vi "Error Converter (ErrCode or Status).vi"(8 "error in (no error)":errorcluster, 11 "error code":i32) -> (0 "error out":errorcluster)   [LabVIEW 2012, in "clearvolume.lvlib"]
uses:
  clearvolume.lvlib
panel:
  in  "string":string="This error is returned by the shared library function."
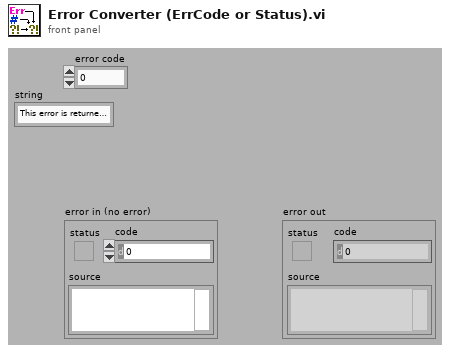
[diagram p1: front panel]
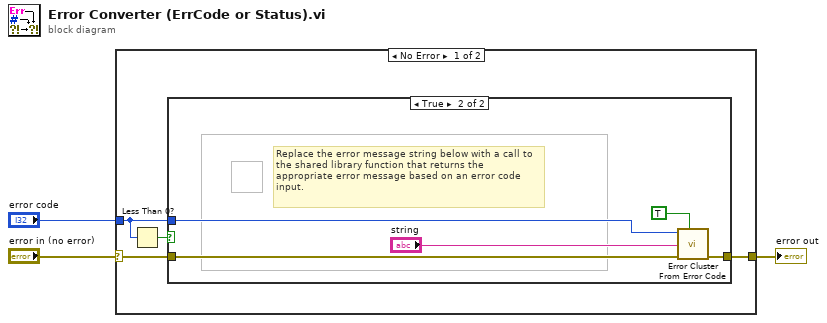
[diagram p0: block diagram]
diagram:
  n1 = case shown="No Error" "error in (no error)" {
    selector: "error in (no error)" -> [w6 w14]
    tunnel: [w4 w14] -> w2
    tunnel: "error code" -> [w5 _]
    frame No Error {
      n2 = Less Than 0?(x=w5) -> (x < 0?=w7:bool)
      n3 = case shown="True" w7 {
        tunnel: w6 -> [w8 w13]
        tunnel: w5 -> [_ w11]
        tunnel: [w8 w12] -> w4
        frame False {
        }
        frame True {
          # "Replace the error message string below with a call to the shared library function that returns the appropriate error message based on an error code input."
          n4 = call <vilib>:"Error Cluster From Error Code.vi"("show call chain? (False)"=TRUE, "error in (no error)"=w13, "error message (\"\")"="string", "error code (0)"=w11) -> ("error out"=w12:errorcluster)  [unwired: 5 in]
        }
      }
    }
    frame Error {
    }
  }
  "error out" <- w2
